vi "Get RelativePath.vi"(8 "error in (no error)":errorcluster caption="错误输入（无错误）", 11 "PanelRootNode 输入":refnum<class "PanelRootNode.lvclass"> caption="DNL_LabVIEW Object in") -> (0 "error out":errorcluster caption="错误输出", 2 "RelativePath":string, 3 "PanelRootNode 输出":refnum<class "PanelRootNode.lvclass"> caption="DNL_LabVIEW Object out")   [LabVIEW 2013, in "PanelRootNode.lvclass"]
uses:
  PanelRootNode.lvclass
  PanelDataNode/PanelDataNode.lvclass/PanelDataNode.ctl
  PanelDataNode/PanelDataNode.lvclass
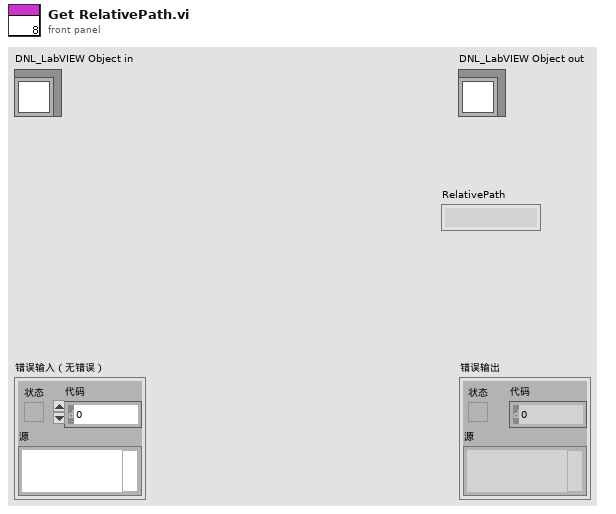
[diagram p1: front panel]
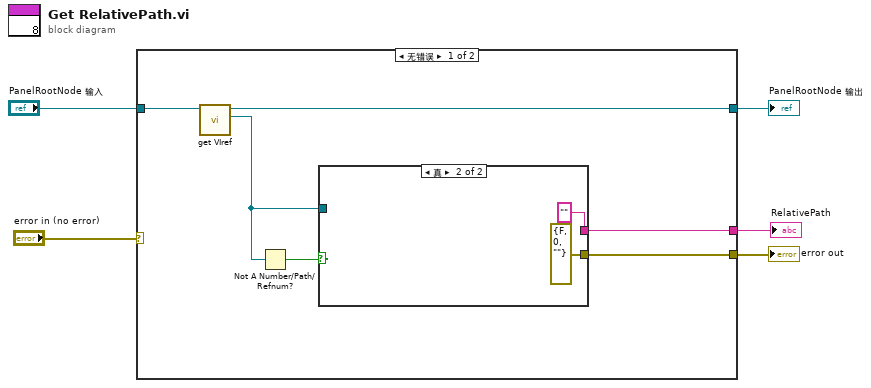
[diagram p0: block diagram]
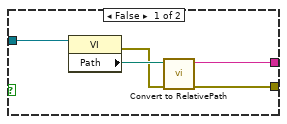
[diagram p2: hidden frame]
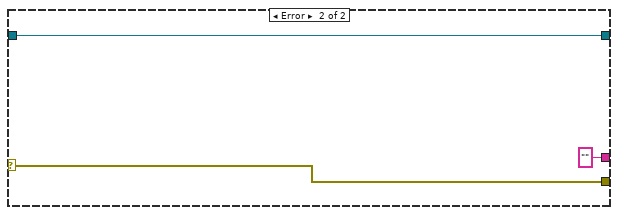
[diagram p3: hidden frame]
diagram:
  n1 = case shown="无错误" "error in (no error)" {
    selector: "error in (no error)" -> [_ w21]
    tunnel: [w6 w21] -> w4
    tunnel: [w10 w20] -> w2
    tunnel: "PanelRootNode 输入" -> [w11 w20]
    tunnel: [w7 "" ("RelativePath")] -> w1
    frame No Error {
      n2 = call "get VIref.vi"("PanelDataNode输入"=w11) -> ("VI*"=w8:refnum<vi>, "PanelDataNode输出"=w10:refnum<class "PanelRootNode.lvclass">)  [unwired: 8 in, 1 out]
      n3 = Not A Number/Path/Refnum?(number/path/refnum=w8) -> (NaN/Path/Refnum?=w9:bool)
      n4 = case shown="真" w9 {
        tunnel: w8 -> [w16 _]
        tunnel: [w14 "" ("RelativePath")] -> w7
        tunnel: [w13 errorcluster {"status"=FALSE, "code"=0, "source"=""} ("error out")] -> w6
        frame False {
          n5 = property class="VI"(reference=w16) -> (error out=w12:errorcluster, "Path"=w15:path)  [unwired: 1 in, 1 out]
          n6 = call "Convert to RelativePath.vi"("error in (no error)"=w12, "VI Path"=w15) -> ("error out"=w13:errorcluster, "RelativePath"=w14:string)  [unwired: 8 in]
        }
        frame True {
        }
      }
    }
    frame Error {
    }
  }
  "error out" <- w4
  "PanelRootNode 输出" <- w2
  "RelativePath" <- w1
